vi "Status Questionable Query.vi"(0 "VISA resource name":refnum<visa-resource-name>, 7 "Query Reg  (0:Summary Enable)":u8(slide) scale=0.0..2.0, 11 "error in (no error)":errorcluster) -> (4 "VISA resource name out":refnum<visa-resource-name>, 8 "SQER (All F:Disable)":bool[](array[boolean]), 15 "error out":errorcluster)   [LabVIEW 2015, in "Chroma ATE 6310.lvlib"]
doc: "The VI returns the setting of selected register in the Status Questionable register group.\n\nThe Questionable Status registers offer you one or more questionable status conditions,which indicate certain errors or faults have occurred on at least one channel."
uses:
  <instrlib>/Chroma ATE 6310/Chroma ATE 6310.lvlib
panel:
  # "CE                VE                 PE                 RV                TE"
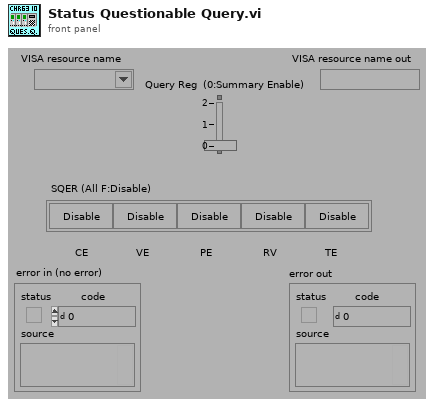
[diagram p1: front panel]
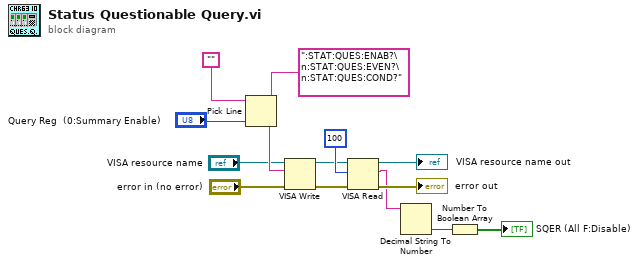
[diagram p0: block diagram]
diagram:
  n1 = Pick Line(string ("")="", multi-line string=":STAT:QUES:ENAB?\n:STAT:QUES:EVEN?\n:STAT:QUES:COND?", line index="Query Reg  (0:Summary Enable)") -> (output string=w9:string)
  n2 = VISA Write(VISA resource name="VISA resource name", write buffer=w9, error in (no error)="error in (no error)") -> (VISA resource name out=w12:refnum<visa-resource-name>, error out=w11:errorcluster)  [unwired: 1 out]
  n3 = VISA Read(VISA resource name=w12, byte count=100, error in (no error)=w11) -> (VISA resource name out=→"VISA resource name out":refnum<visa-resource-name>, read buffer=w1:string, error out=→"error out":errorcluster)  [unwired: 1 out]
  n4 = Decimal String To Number(string=w1) -> (number=w14:i32)  [unwired: 2 in, 1 out]
  n5 = Number To Boolean Array(number=w14) -> (Boolean array=→"SQER (All F:Disable)":bool[])
